vi "gage_pressure.vi"(1 "Atmospheric Pressure [Pa]":dbl, 2 "Abs. Pressure\nVoltage [V]":dbl) -> (0 "Absolute Pressure [Pa]":dbl)   [LabVIEW 2017]
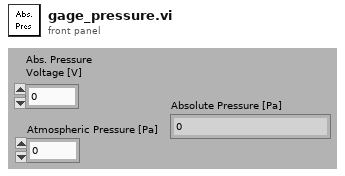
[diagram p1: front panel]
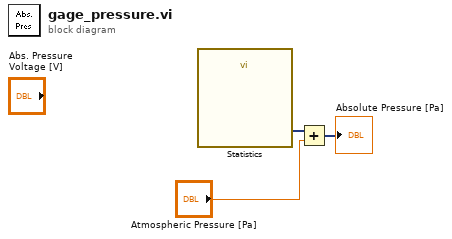
[diagram p0: block diagram]
diagram:
  n1 = call "Statistics"() -> ("Signals"=w5:dynamicdata, "Arithmetic Mean"=w2:dynamicdata)  [unwired: 25 in, 1 out]
  n2 = Add(x=w2, y="Atmospheric Pressure [Pa]") -> (x+y=→"Absolute Pressure [Pa]":dynamicdata)
